vi "pyCode appendNewData.vi"(8 "error in (no error)":errorcluster, 10 "dataArray":string[](array[string]), 11 "pyCode in":refnum<class "pyCode.lvclass">) -> (0 "error out":errorcluster, 3 "pyCode out":refnum<class "pyCode.lvclass">)   [LabVIEW 2018, in "pyCode.lvclass"]
uses:
  pyCode.lvclass
panel:
  out "return value":string
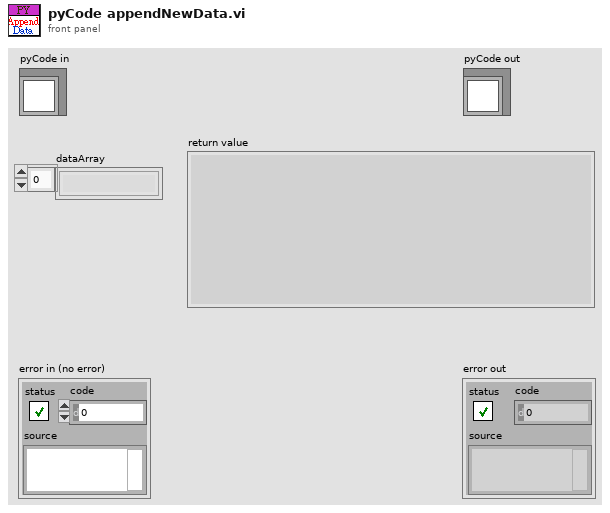
[diagram p1: front panel]
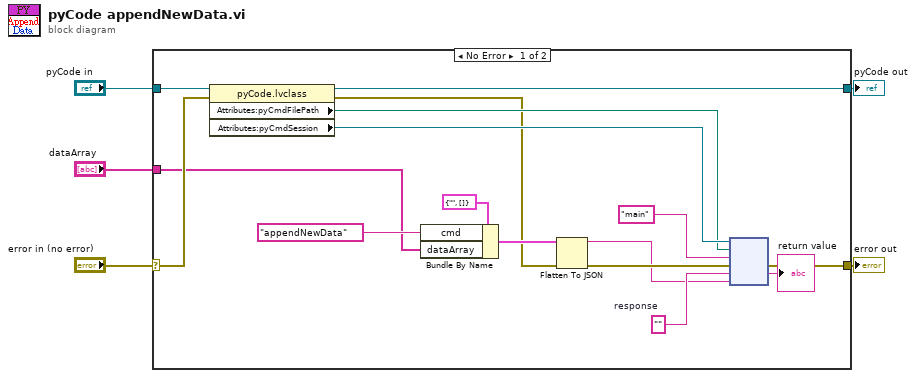
[diagram p0: block diagram]
diagram:
  n1 = case shown="No Error" "error in (no error)" {
    selector: "error in (no error)" -> [w12 w23]
    tunnel: [w10 w23] -> w3
    tunnel: [w20 w22] -> w4
    tunnel: "pyCode in" -> [w21 w22]
    tunnel: "dataArray" -> [w8 _]
    frame No Error {
      w16 = ""  # response
      n2 = property class="pyCode.lvclass"(reference=w21, error in=w12) -> (reference out=w20:refnum<class "pyCode.lvclass">, error out=w11:errorcluster, "Attributes:pyCmdFilePath"=w18:path, "Attributes:pyCmdSession"=w19:refnum<k35>)
      n3 = Bundle By Name(cluster=cluster{"cmd":string, "dataArray":string[]} {"cmd"="", "dataArray"=[]}, "cmd"="appendNewData", "dataArray"=w8) -> (w14:cluster{"cmd":string, "dataArray":string[]})
      n4 = Flatten To JSON(anything=w14, error in (no error)=w11) -> (JSON string=w6:string, 11:w13:errorcluster)  [unwired: 1 in]
      n5 = node(w19, w18, "main" ("function name"), w13, w16, w6) -> (w10:errorcluster, →"return value":string)  [unwired: 1 in, 3 out]
    }
    frame Error {
    }
  }
  "error out" <- w3
  "pyCode out" <- w4
